vi "Set Configuration ID.vi"(8 "error in (no error)":errorcluster, 10 "Configuration ID":i32, 11 "Item Ref in":T1 format="%.0x") -> (0 "error out":errorcluster, 3 "Item Ref out":T1 format="%.0x")   [LabVIEW 2019, in "DSF System Explorer.lvlib"]
uses:
  DSF System Explorer.lvlib
  <vilib>/NI VeriStand/Custom Device API/Custom Device Item Ref.ctl
  <vilib>/NI VeriStand/Custom Device API/Set Item Property (I32).vi
  <vilib>/NI VeriStand/Custom Device API/Custom Device API.lvlib
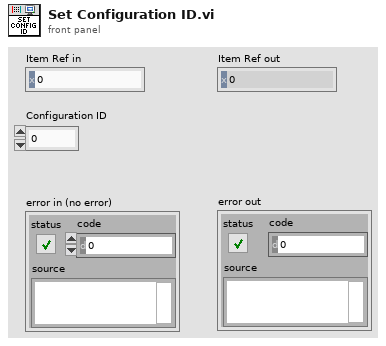
[diagram p1: front panel]
types:
  T1 = typedef "Custom Device API.lvlib/Custom Device Item Ref.ctl" = u64
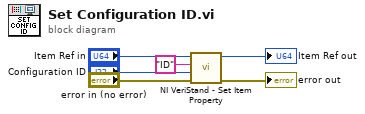
[diagram p0: block diagram]
diagram:
  n1 = call-poly <vilib>:"NI VeriStand - Set Item Property.vi"("error in (no error)"="error in (no error)", "Value"="Configuration ID", "Property Name"="ID", "Item Ref in"="Item Ref in") -> ("error out"=→"error out":errorcluster, "Item Ref out"=→"Item Ref out":T1)  [unwired: 5 in, 1 out]
